vi "Check Status.vi"(8 "error in (no error)":errorcluster, 11 "Function Generator in":refnum<class "Function Generator.lvclass">) -> (0 "error out":errorcluster, 1 "Status":string, 2 "Ready?":bool, 3 "Function Generator out":refnum<class "Function Generator.lvclass">)   [LabVIEW 2015, in "Function Generator.lvclass"]
doc: "Checks if the instrument is powered on and updates its member data with the instrument's current status."
uses:
  Function Generator.lvclass
  FG Channel Settings.ctl
  Tektronix AFG 3000 Series/controls.llb/Waveform Shape.ctl
  Tektronix AFG 3000 Series/controls.llb/Sweep Spacing.ctl
  Tektronix AFG 3000 Series/controls.llb/Sweep Time Parameter.ctl
  Tektronix AFG 3000 Series/controls.llb/Sweep Frequency.ctl
  Tektronix AFG 3000 Series/controls.llb/Voltage.ctl
  Function Generator.lvclass/Function Generator.ctl
  Utility Classes/Scannable/Scannable.lvclass
  Tektronix AFG 3000 Series/Tektronix AFG 3000 Series.lvlib
panel:
  in  "Channel Settings":T1={"General Settings"={" Frequency"=0.0, " Phase"=0.0, " Run Mode"=0, " Waveform Shape"=0, "Output on?"=FALSE}, "Voltage Settings"={"Amplitude"=0.0, "Offset"=0.0}, "Ramp Settings"={"Ramp Symmetry (%)"=50.0}, "Pulse Settings"={"Leading Edge Time "=5e-09, "Trailing Edge Time"=5e-09, "Duty Cycle (%)"=50.0}, "Sweep Mode Settings"={"Start Freq. "=0.0, "Stop Freq.  "=0.0, "Sweep spacing"=0, "Sweep time"=0.0, "Hold time"=0.0, "Return time"=0.0}, "Burst Mode Settings"={"Burst Mode "=1, "Burst Count"=5}, "AM Settings"={"AM Source "=0, "Modulation Waveform "=0, "Modulation Frequency "=1000.0, "Modulation Depth "=0.0}, "FM Settings"={"FM Source "=0, "Modulation Waveform "=0, "Modulation Frequency"=100.0, "Peak Deviation "=100.0}} {"General Settings"."Waveform Shape" items=["Sinusoid", "Square", "Pulse", "Ramp", "PRNoise", "DC", "SINC", "Gaussian", "Lorentz", "ERise", "EDecay", "Haversine", "User 1", "User 2", "User 3", "User 4", "EMemory", "EFile"]; "General Settings"."Run Mode" items=["Continuous", "AM", "FM", "PM", "FSK", "PWM", "Sweep", "Burst"]; "FM Settings"."Modulation Waveform" items=["Sine", "Square", "Triangle", "Ramp", "Down Ramp", "Noise", "User 1", "User 2", "User 3", "User 4", "EMEMory", "EFILe"]; "FM Settings"."FM Source" items=["Internal", "External"]; "AM Settings"."Modulation Waveform" items=["Sine", "Square", "Triangle", "Ramp", "Down Ramp", "Noise"]; "AM Settings"."AM Source" items=["Internal", "External"]; "Burst Mode Settings"."Burst Mode" items=["Triggered", "Gated"]; "Sweep Mode Settings"."Sweep spacing" items=["linear", "log"]; "Pulse Settings"."Trailing Edge Time" format="%#.6g"; "Pulse Settings"."Leading Edge Time" format="%#.6g"; "Ramp Settings"."Ramp Symmetry (%)" min=0.0 max=100.0 step=1.0 format="%.2f"}
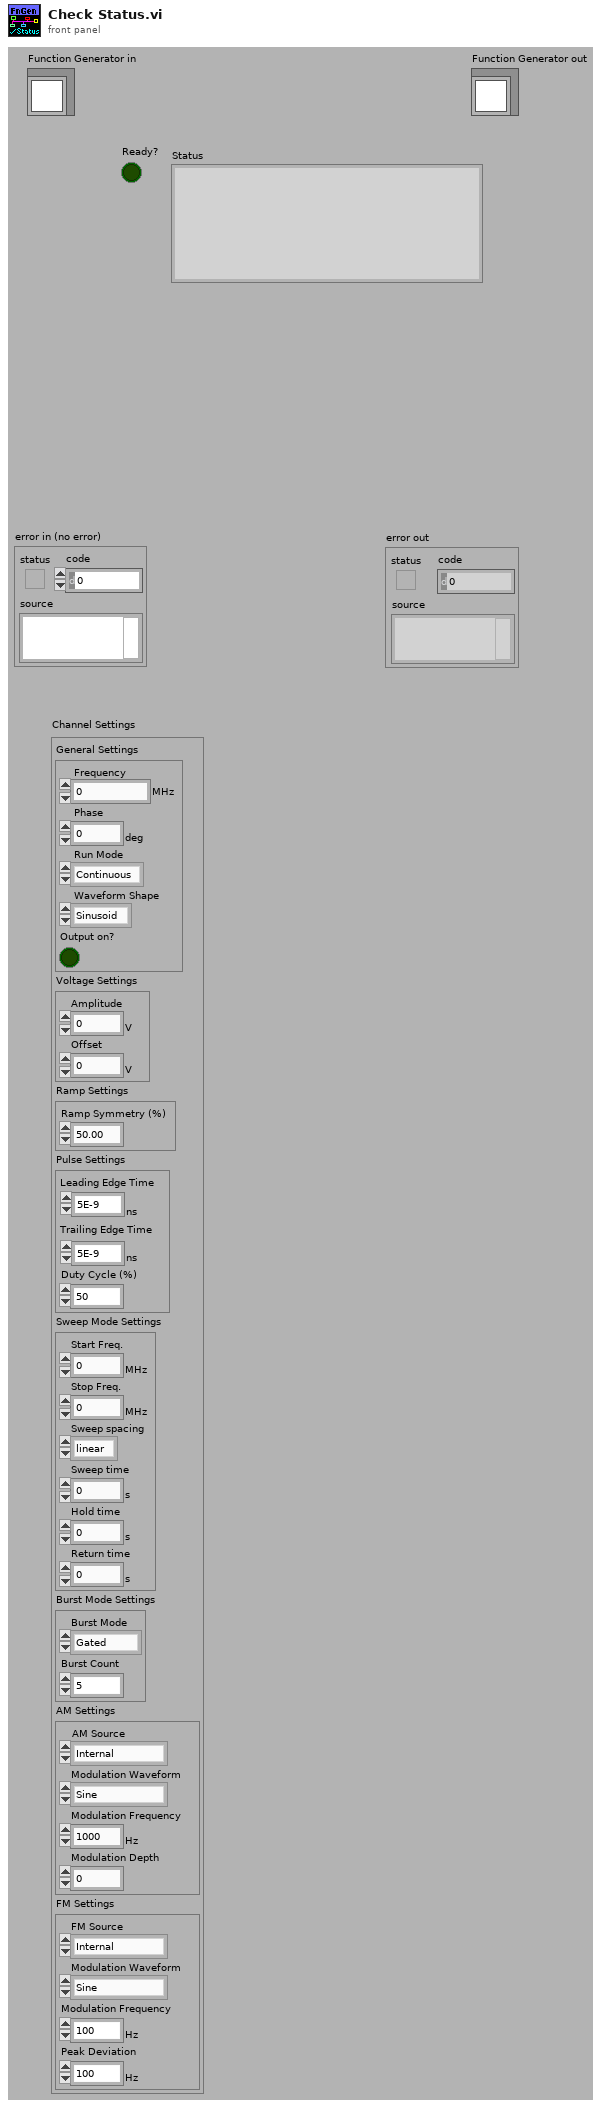
[diagram p1: front panel]
types:
  T1 = typedef "FG Channel Settings.ctl" = cluster{"General Settings":cluster{" Frequency":dbl[unit], " Phase":dbl[unit], " Run Mode":u16, " Waveform Shape":T2, "Output on?":bool}, "Voltage Settings":cluster{"Amplitude":dbl[unit], "Offset":dbl[unit]}, "Ramp Settings":cluster{"Ramp Symmetry (%)":dbl}, "Pulse Settings":cluster{"Leading Edge Time ":dbl[unit], "Trailing Edge Time":dbl[unit], "Duty Cycle (%)":dbl}, "Sweep Mode Settings":cluster{"Start Freq. ":dbl[unit], "Stop Freq.  ":dbl[unit], "Sweep spacing":T3, "Sweep time":dbl[unit], "Hold time":dbl[unit], "Return time":dbl[unit]}, "Burst Mode Settings":cluster{"Burst Mode ":u16, "Burst Count":i32}, "AM Settings":cluster{"AM Source ":u16, "Modulation Waveform ":u16, "Modulation Frequency ":dbl[unit], "Modulation Depth ":dbl}, "FM Settings":cluster{"FM Source ":u16, "Modulation Waveform ":u16, "Modulation Frequency":dbl[unit], "Peak Deviation ":dbl[unit]}}
  T2 = typedef "Waveform Shape.ctl" = u16
  T3 = typedef "Sweep Spacing.ctl" = u16
  T4 = typedef "Voltage.ctl" = enum16{"amplitude", "offset", "high", "low", "high limit", "low limit"}
  T5 = typedef "Sweep Frequency.ctl" = enum16{"center", "span", "start", "stop"}
  T6 = typedef "Sweep Time Parameter.ctl" = enum16{"sweep time", "hold time", "return time"}
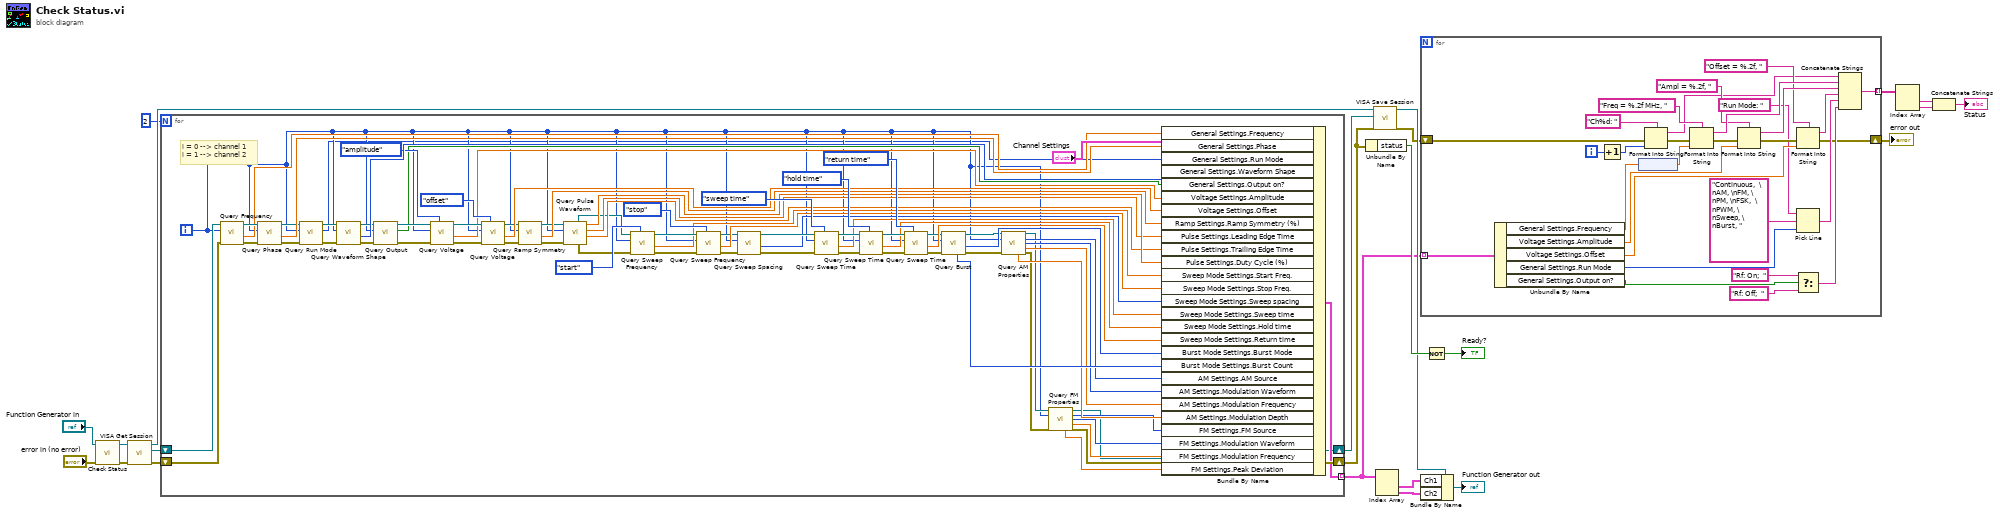
[diagram p0: block diagram]
diagram:
  n1 = call-parent "Check Status.vi"("error in (no error)"="error in (no error)", "Instrument in"="Function Generator in") -> ("error out"=w18:errorcluster, "Instrument out"=w19:refnum<class "Function Generator.lvclass">)  [unwired: 8 out]
  n2 = call-dynamic "VISA Get Session.vi"("error in (no error)"=w18, "Instrument.lvclass in"=w19) -> ("error out"=w17:errorcluster, "VISA Resource Name"=w1:refnum<visa-resource-name>, "Instrument.lvclass out"=w14:refnum<class "Function Generator.lvclass">)  [unwired: 7 out]
  n3 = for {
    N: 2 -> [_]
    shift-right: [w39] -> w15
    shift-left: w17 -> [w89]
    tunnel: [w38] -> w9 mode=indexing
    shift-right: [w37] -> w16
    shift-left: w1 -> [w36]
    i -> [w25]
    # "i = 0 --> channel 1\ni = 1 --> channel 2"
    n4 = call "Query Frequency.vi"("error in (no error)"=w89, "Channel (0: Channel 1)"=w25, "VISA resource name"=w36) -> ("error out"=w88:errorcluster, "frequency"=w86:dbl[unit], "VISA resource name out"=w95:refnum<visa-resource-name>)  [unwired: 6 out]
    n5 = call "Query Phase.vi"("error in (no error)"=w88, "Channel (0: Channel 1)"=w25, "VISA resource name"=w95) -> ("error out"=w27:errorcluster, "phase"=w85:dbl[unit], "VISA resource name out"=w29:refnum<visa-resource-name>)  [unwired: 6 out]
    n6 = call "Query Run Mode.vi"("error in (no error)"=w27, "Channel (0: Channel 1)"=w25, "VISA resource name"=w29) -> ("error out"=w26:errorcluster, "Run Mode"=w24:u16, "VISA resource name out"=w28:refnum<visa-resource-name>)  [unwired: 6 out]
    n7 = call "Query Waveform Shape.vi"("error in (no error)"=w26, "Channel (0: Channel 1)"=w25, "VISA resource name"=w28) -> ("error out"=w32:errorcluster, "Waveform Shape"=w84:T2, "VISA resource name out"=w34:refnum<visa-resource-name>)  [unwired: 6 out]
    n8 = call "Query Output.vi"("error in (no error)"=w32, "Channel (0: Channel 1)"=w25, "VISA resource name"=w34) -> ("error out"=w31:errorcluster, "Output Enabled?"=w30:bool, "VISA resource name out"=w33:refnum<visa-resource-name>)  [unwired: 6 out]
    n9 = call "Query Voltage.vi"("Voltage Param (amplitude)"=Voltage."amplitude", "error in (no error)"=w31, "Channel (0: Channel 1)"=w25, "VISA resource name"=w33) -> ("error out"=w51:errorcluster, "voltage"=w35:dbl[unit], "VISA resource name out"=w81:refnum<visa-resource-name>)  [unwired: 5 out]
    n10 = call "Query Voltage.vi"("Voltage Param (amplitude)"=Voltage."offset", "error in (no error)"=w51, "Channel (0: Channel 1)"=w25, "VISA resource name"=w81) -> ("error out"=w50:errorcluster, "voltage"=w80:dbl[unit], "VISA resource name out"=w79:refnum<visa-resource-name>)  [unwired: 5 out]
    n11 = call "Query Ramp Symmetry.vi"("error in (no error)"=w50, "Channel (0: Channel 1)"=w25, "VISA resource name"=w79) -> ("error out"=w49:errorcluster, "Symmetry (%)"=w78:dbl, "VISA resource name out"=w77:refnum<visa-resource-name>)  [unwired: 6 out]
    n12 = call "Query Pulse Waveform.vi"("error in (no error)"=w49, "Channel (0: Channel 1)"=w25, "VISA resource name"=w77) -> ("Trailing"=w74:dbl[unit], "Leading"=w75:dbl[unit], "Duty Cycle"=w76:dbl, "error out"=w48:errorcluster, "VISA resource name out"=w73:refnum<visa-resource-name>)  [unwired: 4 out]
    n13 = call "Query Sweep Frequency.vi"("Sweep Frequency"=Sweep_Frequency."start", "error in (no error)"=w48, "Channel (0: Channel 1)"=w25, "VISA resource name"=w73) -> ("error out"=w47:errorcluster, "frequency"=w72:dbl[unit], "VISA resource name out"=w98:refnum<visa-resource-name>)  [unwired: 5 out]
    n14 = call "Query Sweep Frequency.vi"("Sweep Frequency"=Sweep_Frequency."stop", "error in (no error)"=w47, "Channel (0: Channel 1)"=w25, "VISA resource name"=w98) -> ("error out"=w46:errorcluster, "frequency"=w71:dbl[unit], "VISA resource name out"=w70:refnum<visa-resource-name>)  [unwired: 5 out]
    n15 = call "Query Sweep Spacing.vi"("error in (no error)"=w46, "Channel (0: Channel 1)"=w25, "VISA resource name"=w70) -> ("error out"=w45:errorcluster, "Sweep spacing (linear)"=w68:T3, "VISA resource name out"=w69:refnum<visa-resource-name>)  [unwired: 6 out]
    n16 = call "Query Sweep Time.vi"("Sweep Time Param (sweep time)"=Sweep_Time_Parameter."sweep time", "error in (no error)"=w45, "Channel (0: Channel 1)"=w25, "VISA resource name"=w69) -> ("error out"=w44:errorcluster, "time"=w67:dbl[unit], "VISA resource name out"=w96:refnum<visa-resource-name>)  [unwired: 5 out]
    n17 = call "Query Sweep Time.vi"("Sweep Time Param (sweep time)"=Sweep_Time_Parameter."hold time", "error in (no error)"=w44, "Channel (0: Channel 1)"=w25, "VISA resource name"=w96) -> ("error out"=w43:errorcluster, "time"=w66:dbl[unit], "VISA resource name out"=w97:refnum<visa-resource-name>)  [unwired: 5 out]
    n18 = call "Query Sweep Time.vi"("Sweep Time Param (sweep time)"=Sweep_Time_Parameter."return time", "error in (no error)"=w43, "Channel (0: Channel 1)"=w25, "VISA resource name"=w97) -> ("error out"=w42:errorcluster, "time"=w65:dbl[unit], "VISA resource name out"=w64:refnum<visa-resource-name>)  [unwired: 5 out]
    n19 = call "Query Burst.vi"("error in (no error)"=w42, "Channel (0: Channel 1)"=w25, "VISA resource name"=w64) -> ("error out"=w41:errorcluster, "Burst Mode"=w63:u16, "VISA resource name out"=w61:refnum<visa-resource-name>, "Burst Count"=w62:i32)  [unwired: 5 out]
    n20 = call "Query AM Properties.vi"("VISA resource name"=w61, "Channel (0: Channel 1)"=w25, "error in (no error)"=w41) -> ("VISA resource name out"=w56:refnum<visa-resource-name>, "AM Source"=w60:u16, "Modulation Waveform"=w59:u16, "Modulation Frequency"=w58:dbl[unit], "Modulation Depth"=w57:dbl, "error out"=w40:errorcluster)  [unwired: 7 out]
    n21 = call "Query FM Properties.vi"("VISA resource name"=w56, "Channel (0: Channel 1)"=w25, "error in (no error)"=w40) -> ("VISA resource name out"=w37:refnum<visa-resource-name>, "FM Source"=w55:u16, "Modulation Waveform"=w54:u16, "Modulation Frequency"=w53:dbl[unit], "Peak Deviation"=w52:dbl[unit], "error out"=w39:errorcluster)  [unwired: 7 out]
    n22 = Bundle By Name(cluster="Channel Settings", "General Settings.Frequency"=w86, "General Settings.Phase"=w85, "General Settings.Run Mode"=w24, "General Settings.Waveform Shape"=w84, "General Settings.Output on?"=w30, "Voltage Settings.Amplitude"=w35, "Voltage Settings.Offset"=w80, "Ramp Settings.Ramp Symmetry (%)"=w78, "Pulse Settings.Leading Edge Time"=w75, "Pulse Settings.Trailing Edge Time"=w74, "Pulse Settings.Duty Cycle (%)"=w76, "Sweep Mode Settings.Start Freq."=w72, "Sweep Mode Settings.Stop Freq."=w71, "Sweep Mode Settings.Sweep spacing"=w68, "Sweep Mode Settings.Sweep time"=w67, "Sweep Mode Settings.Hold time"=w66, "Sweep Mode Settings.Return time"=w65, "Burst Mode Settings.Burst Mode"=w63, "Burst Mode Settings.Burst Count"=w62, "AM Settings.AM Source"=w60, "AM Settings.Modulation Waveform"=w59, "AM Settings.Modulation Frequency"=w58, "AM Settings.Modulation Depth"=w57, "FM Settings.FM Source"=w55, "FM Settings.Modulation Waveform"=w54, "FM Settings.Modulation Frequency"=w53, "FM Settings.Peak Deviation"=w52) -> (w38:T1)
  }
  n23 = Unbundle By Name(w15) -> ("status"=w21:bool)
  n24 = call-dynamic "VISA Save Session.vi"("error in (no error)"=w15, "VISA Resource Name"=w16, "Instrument.lvclass in"=w14) -> ("error out"=w7:errorcluster, "Instrument.lvclass out"=w12:refnum<class "Function Generator.lvclass">)  [unwired: 7 out]
  n25 = Index Array(array=w9) -> (element #1=w10:T1, element #2=w13:T1)  [unwired: 2 in]
  n26 = Bundle By Name(cluster=w12, "Ch1"=w10, "Ch2"=w13) -> (→"Function Generator out":refnum<class "Function Generator.lvclass">)
  n27 = for {
    tunnel: w9 -> [w110] mode=indexing
    shift-right: [w104] -> w8
    shift-left: w7 -> [w103]
    tunnel: [w102] -> w6 mode=indexing
    i -> [w109]
    n28 = Unbundle By Name(w110) -> ("General Settings.Frequency"=w127:dbl[unit], "Voltage Settings.Amplitude"=w125:dbl[unit], "Voltage Settings.Offset"=w124:dbl[unit], "General Settings.Run Mode"=w123:u16, "General Settings.Output on?"=w122:bool)
    n29 = Increment(x=w109) -> (x+1=w99:i32)
    n30 = node(w127) -> (w126:dbl)
    n31 = Format Into String(format string="Ch%d: " ("string (\"\")"), error in=w103, w99) -> (resulting string=w101:string, error out=w107:errorcluster)  [unwired: 1 in]
    n32 = Format Into String(format string="Freq = %.2f MHz, " ("string (\"\")"), error in=w107, w126) -> (resulting string=w118:string, error out=w106:errorcluster)  [unwired: 1 in]
    n33 = Format Into String(format string="Ampl = %.2f, " ("string (\"\")"), error in=w106, w125) -> (resulting string=w115:string, error out=w105:errorcluster)  [unwired: 1 in]
    n34 = Format Into String(format string="Offset = %.2f, " ("string (\"\")"), error in=w105, w124) -> (resulting string=w113:string, error out=w104:errorcluster)  [unwired: 1 in]
    n35 = Pick Line(string ("")="Run Mode: ", multi-line string="Continuous,  \nAM, \nFM, \nPM, \nFSK,  \nPWM, \nSweep, \nBurst, ", line index=w123) -> (output string=w111:string)
    n36 = Select(t="Rf: On;  " ("string (\"\")"), s=w122, f="Rf: Off;  " ("string (\"\")")) -> (s? t:f=w112:string)
    n37 = Concatenate Strings(w101, w118, w115, w113, w111, w112) -> (w102:string)
  }
  "error out" <- w8
  n38 = Not(x=w21) -> (.not. x?=→"Ready?":bool)
  n39 = Index Array(array=w6) -> (element #1=w5:string, element #2=w4:string)  [unwired: 2 in]
  n40 = Concatenate Strings(w5, w4) -> (→"Status":string)
